vi "Parallel exec.vi"(0 "Lower Bound":u32, 5 "Upper Bound":u32=100, 7 "Moving average":dbl=2.0, 8 "Stop":bool, 11 "Error in":errorcluster) -> (15 "Error out":errorcluster)   [LabVIEW 2020]
doc: "This VI is used to executue three VIs parallely in whihc on subVI will generate data and another subVI will generate moving average and plot the data and the third VI is used for documentation purposes."
uses:
  Typedefs/operation numeric lv2.ctl
  Assignment backups/Assignment07 1/Assignment07/Generate and Acquire/Typedefs/Stop cases.ctl
panel:
  in  "File path":path
  out "Generated Number":u32
  in  "File size":i64=100
  out "Moving Avg":dbl[](graph)
  # "PARALLEL EXECUTION"
  # "Bytes"
  # "OUTPUT"
  # "INPUT"
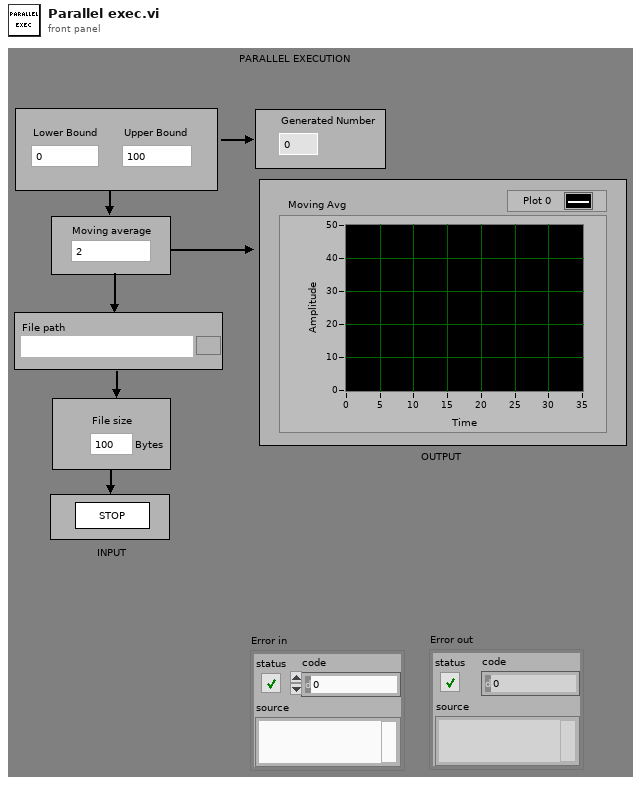
[diagram p1: front panel]
types:
  T1 = typedef "Stop cases.ctl" = enum16{"Initialize", "Write", "Read"}
  T2 = typedef "operation numeric lv2.ctl" = enum16{"Initialize", "Read", "Write", ""}
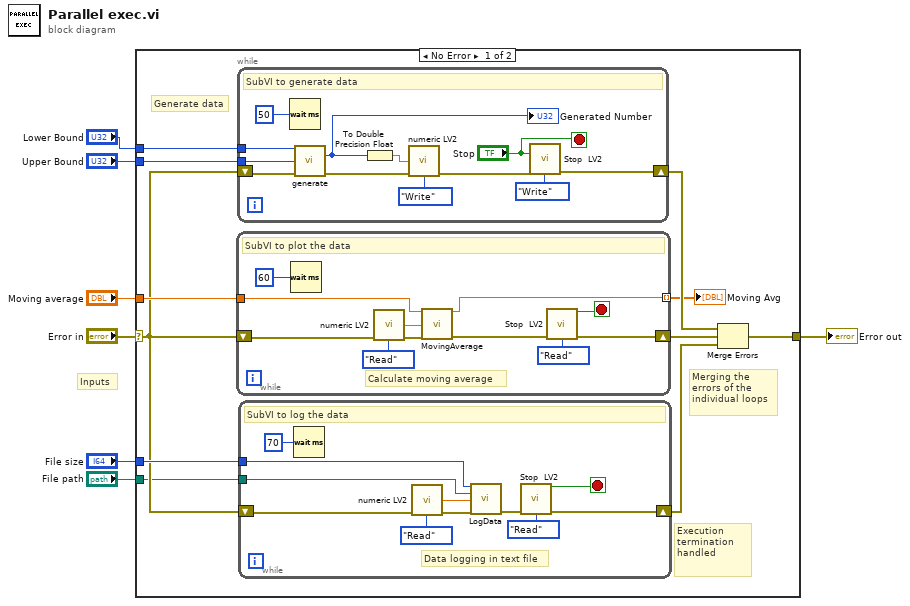
[diagram p0: block diagram]
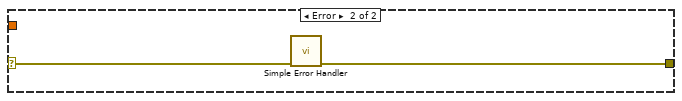
[diagram p2: hidden frame]
diagram:
  # "Inputs"
  n1 = case shown="No Error" "Error in" {
    selector: "Error in" -> [w9 w54]
    tunnel: "Lower Bound" -> [w18 _]
    tunnel: "Upper Bound" -> [w17 _]
    tunnel: [w15 w53] -> w4
    tunnel: "Moving average" -> [w12 _]
    tunnel: "File size" -> [w10 _]
    tunnel: "File path" -> [w8 _]
    frame No Error {
      # "Execution termination\nhandled"
      # "Generate data"
      # "Merging the \nerrors of the \nindividual loops"
      n2 = while {
        tunnel: w12 -> [w37]
        tunnel: [w36] -> w11 mode=indexing
        shift-right: [w39] -> w14
        shift-left: w9 -> [w38]
        stop <- w40 stop-if-true
        # "Calculate moving average"
        # "SubVI to plot the data"
        n3 = Wait (ms)(milliseconds to wait=u32 60) -> ()  [unwired: 1 out]
        n4 = call "numeric LV2.vi"("Error in"=w38, "Operation"=operation_numeric_lv2."Read") -> ("Numeric out"=w33:dbl, "Error out"=w35:errorcluster)  [unwired: 12 in]
        n5 = call "MovingAverage.vi"("Moving average"=w37, "Random number"=w33, "Error in"=w35) -> ("Average"=w36:dbl, "Error out"=w34:errorcluster)  [unwired: 11 in]
        n6 = call "Stop  LV2.vi"("Error in"=w34, "Operation"=Stop_cases."Read") -> ("Output"=w40:bool, "Error out"=w39:errorcluster)  [unwired: 12 in]
      }
      "Moving Avg" <- w11
      n7 = while {
        tunnel: w18 -> [w49]
        tunnel: w17 -> [w48]
        shift-right: [w50] -> w16
        shift-left: w9 -> [w51]
        stop <- "Stop" stop-if-true
        # "SubVI to generate data"
        n8 = Wait (ms)(milliseconds to wait=u32 50) -> ()  [unwired: 1 out]
        n9 = call "generate.vi"("lower bound"=w49, "upper bound"=w48, "Error in"=w51) -> ("Generated number"=w47:u32, "Error out"=w46:errorcluster)  [unwired: 11 in]
        "Generated Number" <- w47
        n10 = To Double Precision Float(number=w47) -> (double precision float=w45:dbl)
        n11 = call "numeric LV2.vi"("Numeric in"=w45, "Error in"=w46, "Operation"=operation_numeric_lv2."Write") -> ("Error out"=w44:errorcluster)  [unwired: 11 in, 1 out]
        n12 = call "Stop  LV2.vi"("Stop"="Stop", "Error in"=w44, "Operation"=Stop_cases."Write") -> ("Error out"=w50:errorcluster)  [unwired: 11 in, 1 out]
      }
      n13 = while {
        tunnel: w10 -> [w27]
        tunnel: w8 -> [w25]
        shift-right: [w28] -> w13
        shift-left: w9 -> [w26]
        stop <- w29 stop-if-true
        # "Data logging in text file"
        # "SubVI to log the data"
        n14 = Wait (ms)(milliseconds to wait=u32 70) -> ()  [unwired: 1 out]
        n15 = call "numeric LV2.vi"("Error in"=w26, "Operation"=operation_numeric_lv2."Read") -> ("Numeric out"=w23:dbl, "Error out"=w24:errorcluster)  [unwired: 12 in]
        n16 = call "LogData.vi"("file size"=w27, "File path"=w25, "Numeric"=w23, "Error in"=w24) -> ("Error out"=w22:errorcluster)  [unwired: 11 in]
        n17 = call "Stop  LV2.vi"("Error in"=w22, "Operation"=Stop_cases."Read") -> ("Output"=w29:bool, "Error out"=w28:errorcluster)  [unwired: 12 in]
      }
      n18 = Merge Errors(w16, w14, w13) -> (w15:errorcluster)
    }
    frame Error {
      n19 = call <vilib>:"Simple Error Handler.vi"("error in (no error)"=w54) -> ("error out"=w53:errorcluster)  [unwired: 4 in, 4 out]
    }
  }
  "Error out" <- w4
